vi "Set Command FIFO.vi"(10 "command fifo":refnum<k33>, 11 "Interface in":refnum<class "Interface.lvclass">) -> (3 "Interface out":refnum<class "Interface.lvclass">)   [LabVIEW 2020, in "DSF Core.lvlib" / "Interface.lvclass"]
uses:
  Interface.lvclass
  Interface.lvclass/Interface.ctl
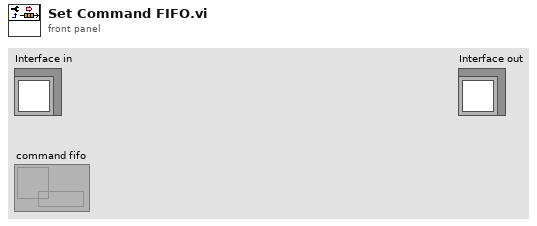
[diagram p1: front panel]
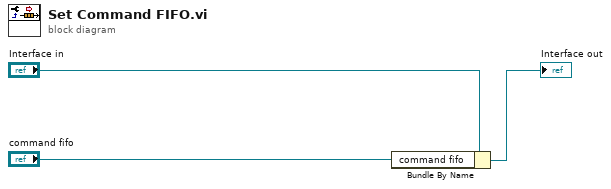
[diagram p0: block diagram]
diagram:
  n1 = Bundle By Name(cluster="Interface in", "command fifo"="command fifo") -> (→"Interface out":refnum<class "Interface.lvclass">)
